vi "Pitch.vi"(5 "input":path, 7 "Pitch":dbl) -> (6 "output":path)   [LabVIEW 2012]
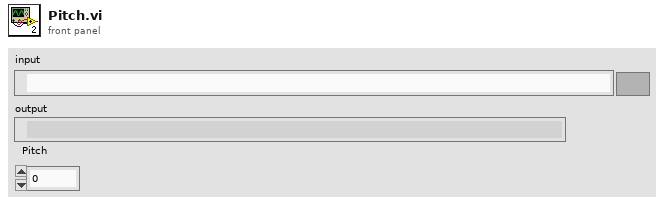
[diagram p1: front panel]
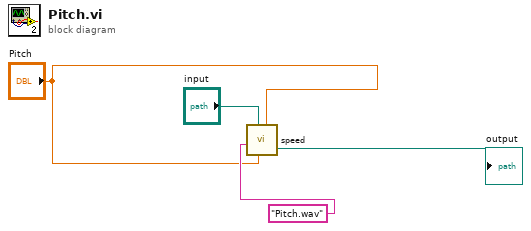
[diagram p0: block diagram]
diagram:
  n1 = call "speed.vi"("speed"="Pitch", "dt Scaling"="Pitch", "input"="input", "replacementString"="Pitch.wav" ("replace string (\"\")")) -> ("output"=→"output":path)  [unwired: 7 in]
